vi "Verify File.vi"(5 "Options":T1, 7 "Test VI (caller)":string, 8 "error in":errorcluster, 10 "path to VI or CTL":path) -> (0 "error out":errorcluster)   [LabVIEW 2020, in "Caraya.Extension.lvlib"]
uses:
  Caraya.Extension.lvlib
  Approval Tests/Options.ctl
  Approval Tests/Reporter/Reporter.lvclass
  Approval Tests/Printer/Printer.lvclass
  <vilib>/addons/_JKI Toolkits/Caraya/classes/Assert/Assert True.vi
  <vilib>/addons/_JKI Toolkits/Caraya/classes/Assert/Assert.lvclass
  Approval Tests/Approval Tests.lvlib
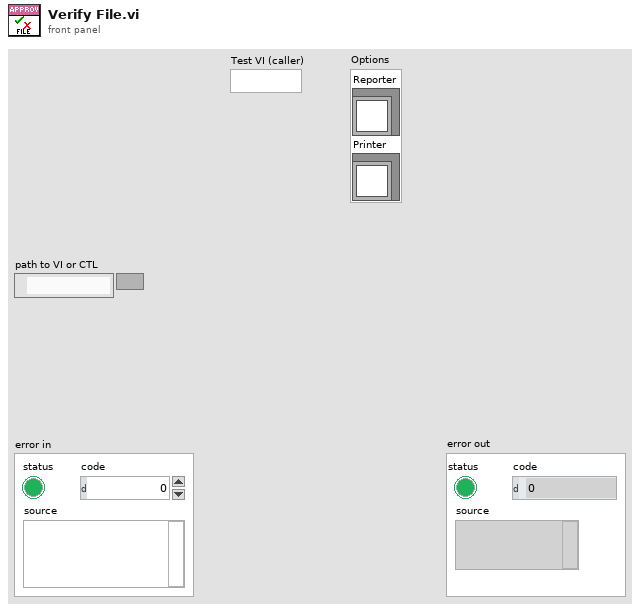
[diagram p1: front panel]
types:
  T1 = typedef "Approval Tests.lvlib/Options.ctl" = cluster{"Reporter":refnum<class "Reporter.lvclass">, "Printer":refnum<class "Printer.lvclass">}
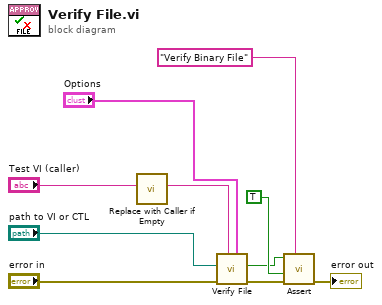
[diagram p0: block diagram]
diagram:
  n1 = call "Replace with Caller if Empty.vi"("Test VI (caller) in"="Test VI (caller)") -> ("Test VI (caller) out"=w2:string)  [unwired: 10 in]
  n2 = call "Verify File.vi"("Options"="Options", "Test VI (caller)"=w2, "error in"="error in", "Path to Binary File to Verify"="path to VI or CTL") -> ("error out"=w6:errorcluster, "Passed?"=w5:bool)  [unwired: 5 in, 1 out]
  n3 = call-poly <vilib>:"Assert.vi"("Label"="Verify Binary File", "error in (no error)"=w6, "Register with caller test (F)"=TRUE, "True?"=w5) -> ("error out"=→"error out":errorcluster)  [unwired: 6 in, 1 out]
